vi "Autônomo.vi"() -> ()   [LabVIEW 2020]
uses:
  <vilib>/Platform/TimedLoop/XDataNode/timing_clust.ctl
  <vilib>/Platform/TimedLoop/XDataNode/nitl_modes.ctl
  <vilib>/Platform/TimedLoop/XDataNode/wakeup.ctl
  <vilib>/Rock Robotics/WPI/ThirdParty/Phoenix-LabVIEW/Motor Controller/Controls/CTRE_Phoenix_MotorControl_ControlMode.ctl
  <vilib>/Rock Robotics/WPI/Utilities/WPI_GetSetVariantRefNum.vi
  <vilib>/Rock Robotics/WPI/RobotDrive/WPI_RobotDriveArcadeDrive_Standard(NoSaturation).vi
  <vilib>/platform/TimedLoop/XDataNode/XDataNode.xnode
  <vilib>/Rock Robotics/Network Tables/NT Write Number.vi
  Prog_Testes/GlobalVariables.vi
  <vilib>/Rock Robotics/Network Tables/NT Write Numeric Array.vi
  <vilib>/Platform/TimedLoop/XDataNode/XDNodeRunTimeDep.lvlib
  <vilib>/Rock Robotics/SystemInterfaces/DIO/FPGA_DIOPWMChannel.ctl
  <vilib>/Rock Robotics/WPI/PWM/WPI_PWMDeadband.ctl
  <vilib>/Rock Robotics/WPI/MotorControl/WPI_MotorControlType.ctl
  <vilib>/Rock Robotics/SystemInterfaces/DIO/FPGA_DIOChannel.ctl
  <vilib>/Rock Robotics/WPI/MotorControl/WPI_MotorControlDeviceRef.ctl
  <vilib>/Rock Robotics/WPI/RobotDrive/WPI_RobotDriveDevRef.ctl
panel:
  out "Vm1":T1={"DevStatus"={"status"=FALSE, "code"=0, "source"=""}, "Motors[]"=[], "Square Inputs"=FALSE, "Max Output"=1.0}
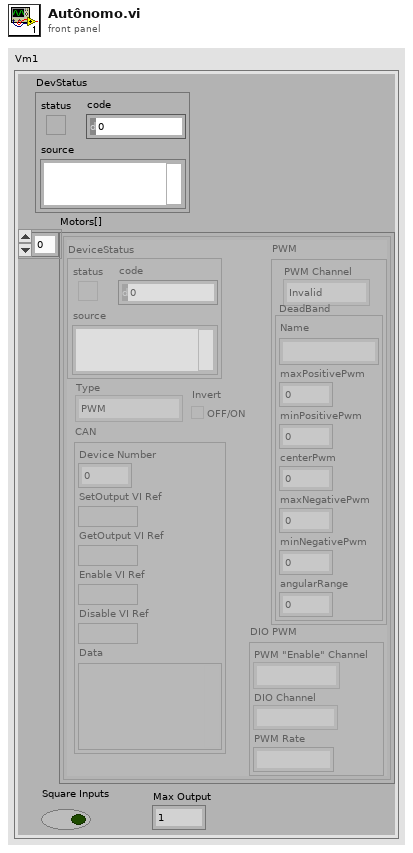
[diagram p1: front panel]
types:
  T1 = typedef "WPI_RobotDriveDevRef.ctl" = cluster{"DevStatus":errorcluster, "Motors[]":T2[], "Square Inputs":bool, "Max Output":dbl}
  T2 = typedef "WPI_MotorControlDeviceRef.ctl" = cluster{"DeviceStatus":errorcluster, "Type":T3, "PWM":cluster{"PWM Channel":T4, "DeadBand":T5}, "CAN":cluster{"Device Number":u8, "SetOutput VI Ref":variant, "GetOutput VI Ref":variant, "Enable VI Ref":variant, "Disable VI Ref":variant, "Data":variant}, "Invert":bool, "DIO PWM":cluster{"PWM \"Enable\" Channel":T4, "DIOChannel":T6, "PWM Rate":dbl}}
  T3 = typedef "WPI_MotorControlType.ctl" = enum16{"PWM", "CAN", "DIO PWM"}
  T4 = typedef "FPGA_DIOPWMChannel.ctl" = enum8{"PWM 0", "PWM 1", "PWM 2", "PWM 3", "PWM 4", "PWM 5", "PWM 6", "PWM 7", "PWM 8", "PWM 9", "PWM MXP 0", "PWM MXP 1", "PWM MXP 2", "PWM MXP 3", "PWM MXP 4", "PWM MXP 5", "PWM MXP 6", "PWM MXP 7", "PWM MXP 8", "PWM MXP 9", "Invalid"}
  T5 = typedef "WPI_PWMDeadband.ctl" = cluster{"Name":string, "maxPositivePwm":i32, "minPositivePwm":i32, "centerPwm":i32, "maxNegativePwm":i32, "minNegativePwm":i32, "angularRange":u16}
  T6 = typedef "FPGA_DIOChannel.ctl" = enum8{"DIO 0", "DIO 1", "DIO 2", "DIO 3", "DIO 4", "DIO 5", "DIO 6", "DIO 7", "DIO 8", "DIO 9", "DIO MXP 0", "DIO MXP 1", "DIO MXP 2", "DIO MXP 3", "DIO MXP 4", "DIO MXP 5", "DIO MXP 6", "DIO MXP 7", "DIO MXP 8", "DIO MXP 9", "DIO MXP 10", "DIO MXP 11", "DIO MXP 12", "DIO MXP 13", "DIO MXP 14", "DIO MXP 15", "SPI Port CS1", "SPI Port CS2", "SPI Port CS3", "SPI Port MISO", "SPI Port MOSI", "Invalid"}
  T7 = typedef "XDNodeRunTimeDep.lvlib/timing_clust.ctl" = cluster{"Expected End [f-1]":u64, "Actual End [f-1]":u64, "Finished Late? [f-1]":bool, "Expected End [i-1]":u64, "Actual End [i-1]":u64, "Finished Late? [i-1]":bool, "Expected Start [i]":u64, "Actual Start [i]":u64, "Expected Start [f]":u64, "Actual Start [f]":u64, "Source Name":string, "Structure Name":string, "Period":i64, "Deadline":i64, "Offset":i64, "Start":i64, "Priority":i32, "Timeout":i32, "Mode":T8, "Wakeup Reason":T9, "Error":errorcluster, "Source Type":string, "Secondary Source Type":string, "Global End Time":u64, "Global Start Time":u64, "Frame Duration":u64, "Iteration Duration":u64, "Assigned CPU":i32, "I/O Scan Engine Mode":u32}
  T8 = typedef "XDNodeRunTimeDep.lvlib/nitl_modes.ctl" = enum32{"No Change", "Process missed periods, maintain original phase", "Discard missed periods, maintain original phase", "Process missed periods, ignore original phase", "Discard missed periods, ignore original phase"}
  T9 = typedef "XDNodeRunTimeDep.lvlib/wakeup.ctl" = enum32{"Normal", "Aborted", "Asynchronous wakeup", "Timing source error", "Timed loop error", "Timeout"}
  T10 = typedef "CTRE_Phoenix_MotorControl_ControlMode.ctl" = u16
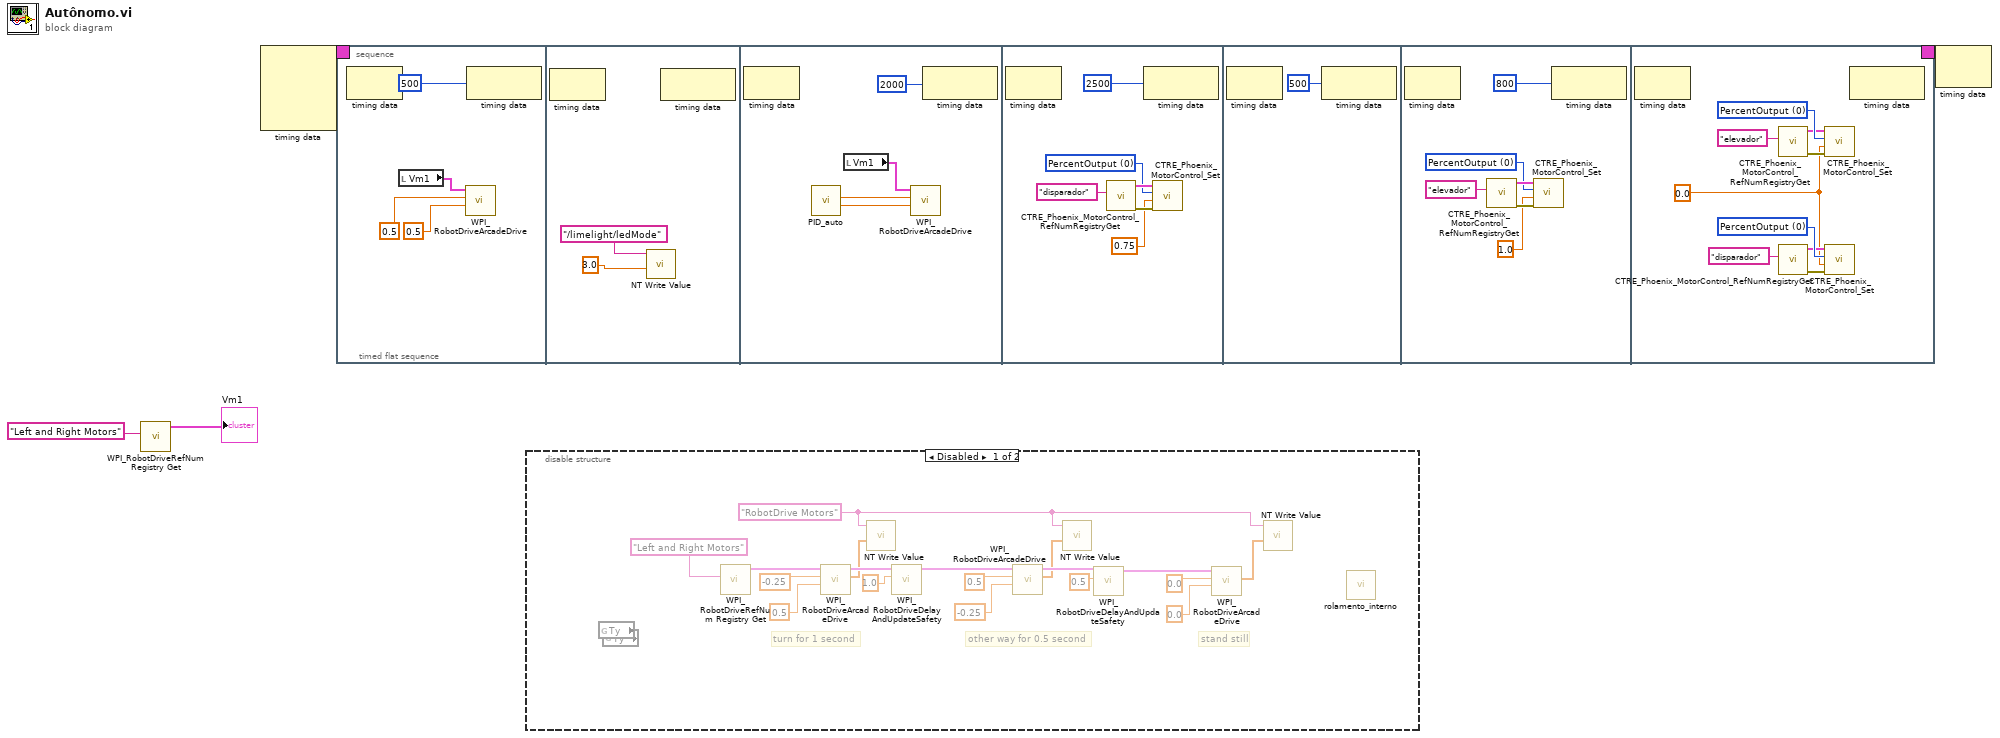
[diagram p0: block diagram]
diagram:
  n1 = call <vilib>:"WPI_RobotDriveRefNum Registry Get.vi"("refnum name"="Left and Right Motors") -> ("RobotDriveDevRef"=→"Vm1":T1)  [unwired: 9 in, 1 out]
  n2 = node-c288() -> (w3:T7)  [unwired: 4 in]
  n3 = timed-sequence {
    timing: w3 -> [_]
    timing-out: [_] -> w2
    n4 = timed-flat-sequence {
      frame #0 {
        n5 = node-c288() -> ()  [unwired: 1 in, 1 out]
        n6 = local read "Vm1"() -> (w5:T1)
        n7 = call-poly <vilib>:"WPI_RobotDriveArcadeDrive.vi"("Y axis value"=0.5 ("X axis value"), "X axis value"=0.5, "RobotDriveDevRef"=w5) -> ()  [unwired: 1 in, 8 out]
        n8 = node-c288(u32 500 ("milliseconds to wait")) -> ()  [unwired: 1 out]
      }
      frame #1 {
        n9 = node-c288() -> ()  [unwired: 1 in, 1 out]
        n10 = call-poly <vilib>:"NT Write Value.vi"("Numeric"=3.0, "Name"="/limelight/ledMode") -> ()  [unwired: 9 in, 1 out]
        n11 = node-c288() -> ()  [unwired: 1 in, 1 out]
      }
      frame #2 {
        n12 = node-c288() -> ()  [unwired: 1 in, 1 out]
        n13 = call "PID_auto.vi"() -> ("output_ty"=w20:dbl, "output_tx"=w19:dbl)  [unwired: 10 in]
        n14 = local read "Vm1"() -> (w17:T1)
        n15 = call-poly <vilib>:"WPI_RobotDriveArcadeDrive.vi"("Y axis value"=w20, "X axis value"=w19, "RobotDriveDevRef"=w17) -> ()  [unwired: 1 in, 8 out]
        n16 = node-c288(u32 2000 ("milliseconds to wait")) -> ()  [unwired: 1 out]
      }
      frame #3 {
        w27 = T10 0 items=["PercentOutput"=0, "Position"=1, "Velocity"=2, "Current"=3, "Follower"=5, "MotionProfile"=6, "MotionMagic"=7, "MotionProfileArc"=10, "Disabled"=15] ("Control Mode")
        n17 = node-c288() -> ()  [unwired: 1 in, 1 out]
        n18 = call <vilib>:"CTRE_Phoenix_MotorControl_RefNumRegistryGet.vi"("refnum name"="disparador") -> ("error out"=w30:errorcluster, "PhoenixMotorControlDevRef"=w29:T2)  [unwired: 9 in]
        n19 = node-c288(u32 2500 ("milliseconds to wait")) -> ()  [unwired: 1 out]
        n20 = call <vilib>:"CTRE_Phoenix_MotorControl_Set.vi"("error in (no error)"=w30, "Output"=0.75, "Control Mode"=w27, "PhoenixMotorControlDevRef"=w29) -> ()  [unwired: 6 in, 2 out]
      }
      frame #4 {
        n21 = node-c288() -> ()  [unwired: 1 in, 1 out]
        n22 = node-c288(u32 500 ("milliseconds to wait")) -> ()  [unwired: 1 out]
      }
      frame #5 {
        w43 = T10 0 items=["PercentOutput"=0, "Position"=1, "Velocity"=2, "Current"=3, "Follower"=5, "MotionProfile"=6, "MotionMagic"=7, "MotionProfileArc"=10, "Disabled"=15] ("Control Mode")
        n23 = node-c288() -> ()  [unwired: 1 in, 1 out]
        n24 = call <vilib>:"CTRE_Phoenix_MotorControl_RefNumRegistryGet.vi"("refnum name"="elevador") -> ("error out"=w45:errorcluster, "PhoenixMotorControlDevRef"=w44:T2)  [unwired: 9 in]
        n25 = call <vilib>:"CTRE_Phoenix_MotorControl_Set.vi"("error in (no error)"=w45, "Output"=1.0, "Control Mode"=w43, "PhoenixMotorControlDevRef"=w44) -> ()  [unwired: 6 in, 2 out]
        n26 = node-c288(u32 800 ("milliseconds to wait")) -> ()  [unwired: 1 out]
      }
      frame #6 {
        w50 = 0.0
        w53 = T10 0 items=["PercentOutput"=0, "Position"=1, "Velocity"=2, "Current"=3, "Follower"=5, "MotionProfile"=6, "MotionMagic"=7, "MotionProfileArc"=10, "Disabled"=15] ("Control Mode")
        w57 = T10 0 items=["PercentOutput"=0, "Position"=1, "Velocity"=2, "Current"=3, "Follower"=5, "MotionProfile"=6, "MotionMagic"=7, "MotionProfileArc"=10, "Disabled"=15] ("Control Mode")
        n27 = node-c288() -> ()  [unwired: 1 in, 1 out]
        n28 = call <vilib>:"CTRE_Phoenix_MotorControl_RefNumRegistryGet.vi"("refnum name"="elevador") -> ("error out"=w55:errorcluster, "PhoenixMotorControlDevRef"=w56:T2)  [unwired: 9 in]
        n29 = call <vilib>:"CTRE_Phoenix_MotorControl_RefNumRegistryGet.vi"("refnum name"="disparador") -> ("error out"=w51:errorcluster, "PhoenixMotorControlDevRef"=w52:T2)  [unwired: 9 in]
        n30 = call <vilib>:"CTRE_Phoenix_MotorControl_Set.vi"("error in (no error)"=w55, "Output"=w50, "Control Mode"=w57, "PhoenixMotorControlDevRef"=w56) -> ()  [unwired: 6 in, 2 out]
        n31 = call <vilib>:"CTRE_Phoenix_MotorControl_Set.vi"("error in (no error)"=w51, "Output"=w50, "Control Mode"=w53, "PhoenixMotorControlDevRef"=w52) -> ()  [unwired: 6 in, 2 out]
        n32 = node-c288() -> ()  [unwired: 1 in, 1 out]
      }
    }
  }
  n33 = disable-structure shown="Disabled" {
    frame Disabled {
      w62 = "RobotDrive Motors" ("Name")
      # "stand still"
      # "other way for 0.5 second"
      # "turn for 1 second"
      n34 = global read "GlobalVariables.vi" "Ty"() -> ()  [unwired: 1 out]
      n35 = global read "GlobalVariables.vi" "Ty"() -> ()  [unwired: 1 out]
      n36 = call <vilib>:"WPI_RobotDriveRefNum Registry Get.vi"("refnum name"="Left and Right Motors") -> ("RobotDriveDevRef"=w78:T1)  [unwired: 1 in, 9 out]
      n37 = call-poly <vilib>:"WPI_RobotDriveArcadeDrive.vi"("Y axis value"=0.5 ("X axis value"), "X axis value"=-0.25, "RobotDriveDevRef"=w78) -> ("Motor Values"=w61:dbl[], "RobotDriveDevRef"=w71:T1)  [unwired: 1 in, 6 out]
      n38 = call-poly <vilib>:"NT Write Value.vi"("Numeric Array"=w61, "Name"=w62) -> ()  [unwired: 9 in, 1 out]
      n39 = call <vilib>:"WPI_RobotDriveDelayAndUpdateSafety.vi"("Delay (s)"=1.0, "RobotDriveDevRef"=w71) -> ("RobotDriveDevRef 2"=w72:T1)  [unwired: 8 in, 1 out]
      n40 = call-poly <vilib>:"WPI_RobotDriveArcadeDrive.vi"("Y axis value"=-0.25 ("X axis value"), "X axis value"=0.5, "RobotDriveDevRef"=w72) -> ("Motor Values"=w63:dbl[], "RobotDriveDevRef"=w73:T1)  [unwired: 1 in, 6 out]
      n41 = call-poly <vilib>:"NT Write Value.vi"("Numeric Array"=w63, "Name"=w62) -> ()  [unwired: 9 in, 1 out]
      n42 = call <vilib>:"WPI_RobotDriveDelayAndUpdateSafety.vi"("Delay (s)"=0.5, "RobotDriveDevRef"=w73) -> ("RobotDriveDevRef 2"=w74:T1)  [unwired: 8 in, 1 out]
      n43 = call-poly <vilib>:"WPI_RobotDriveArcadeDrive.vi"("Y axis value"=0.0 ("X axis value"), "X axis value"=0.0, "RobotDriveDevRef"=w74) -> ("Motor Values"=w64:dbl[])  [unwired: 1 in, 7 out]
      n44 = call-poly <vilib>:"NT Write Value.vi"("Numeric Array"=w64, "Name"=w62) -> ()  [unwired: 9 in, 1 out]
      n45 = call "rolamento_interno.vi"() -> ()  [unwired: 12 in]
    }
    frame Enabled {
    }
  }
  n46 = node-c288(w2) -> ()  [unwired: 1 out]
